vi "Tree_Get nearest top displayed item.vi"(9 "Retained Tags":string[](array[string]), 10 "Original Tags":string[](array[string]), 11 "Top Tag In":string) -> (3 "Top Tag Out":string)   [LabVIEW 2023]
doc: "Find tree tiem nearest to top displayed item that is still available to display after filtering. Used to keep current rree view about the same when filtering on show/hide scripting and private properties."
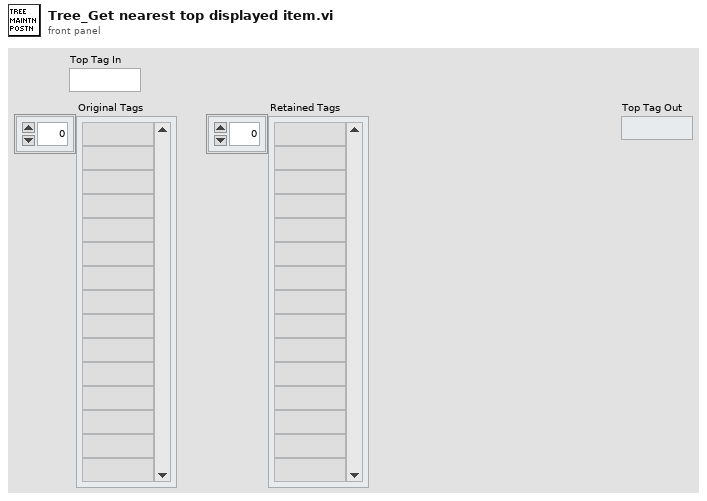
[diagram p1: front panel]
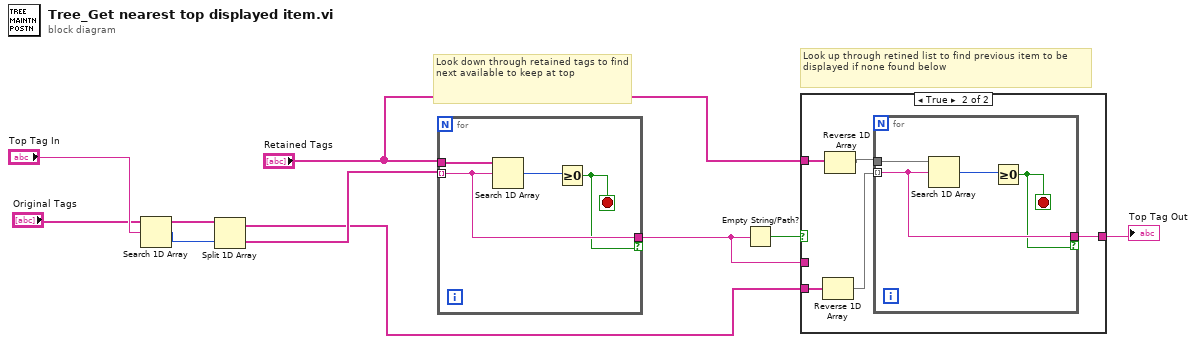
[diagram p0: block diagram]
diagram:
  # "Look up through retined list to find previous item to be displayed if none found below"
  # "Look down through retained tags to find next available to keep at top"
  n1 = Search 1D Array(1D array="Original Tags", element="Top Tag In") -> (index of element=w7:i32)  [unwired: 1 in]
  n2 = Split 1D Array(array="Original Tags", index=w7) -> (first subarray=w3:string[], second subarray=w6:string[])
  n3 = for {
    tunnel: "Retained Tags" -> [w13]
    tunnel: w6 -> [w11] mode=indexing
    tunnel: [w11] -> w1 if=w10
    stop <- w10 stop-if-true
    n4 = Search 1D Array(1D array=w13, element=w11) -> (index of element=w12:i32)  [unwired: 1 in]
    n5 = Greater Or Equal To 0?(x=w12) -> (x >= 0?=w10:bool)
  }
  n6 = Empty String/Path?(string/path=w1) -> (empty?=w5:bool)
  n7 = case shown="True" w5 {
    tunnel: "Retained Tags" -> [_ w19]
    tunnel: w3 -> [_ w17]
    tunnel: [w14 w16] -> w2
    tunnel: w1 -> [w14 _]
    frame False {
    }
    frame True {
      n8 = Reverse 1D Array(array=w17) -> (reversed array=w15:string[])
      n9 = Reverse 1D Array(array=w19) -> (reversed array=w18:string[])
      n10 = for {
        tunnel: w18 -> [w23]
        tunnel: w15 -> [w21] mode=indexing
        tunnel: [w21] -> w16 if=w20
        stop <- w20 stop-if-true
        n11 = Search 1D Array(1D array=w23, element=w21) -> (index of element=w22:i32)  [unwired: 1 in]
        n12 = Greater Or Equal To 0?(x=w22) -> (x >= 0?=w20:bool)
      }
    }
  }
  "Top Tag Out" <- w2
